vi "Output Enable Write Single.vi"() -> ()   [LabVIEW 2023, in "Output Enable.lvclass"]
uses:
  Output Enable.lvclass
  Output Enable.lvclass/Output Enable.ctl
  <vilib>/ADAS Replay HIL/Channels/Tag Wrapper/Tag Wrapper.lvlib
  <vilib>/ADAS Replay HIL/Channels/Tag Wrapper/Polymorphic/Write Channel (I32).vi
panel:
  in  "Timeout (ms)":i32
  in  "Value to Write":i32
  out "Output Enable out":refnum<class "Output Enable.lvclass">
  in  "Output Enable in":refnum<class "Output Enable.lvclass">
  in  "Channel Index":i32=1
  out "error out":errorcluster
  in  "error in":errorcluster
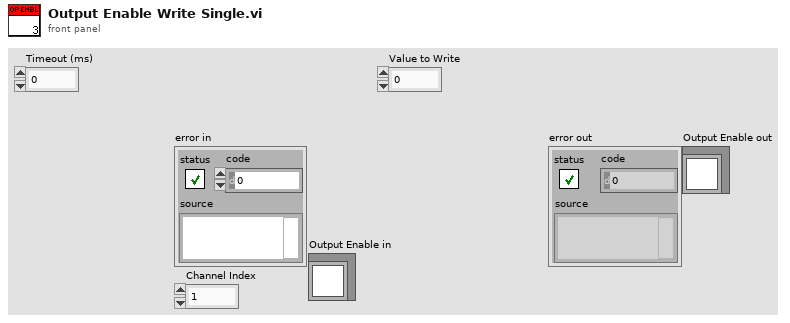
[diagram p1: front panel]
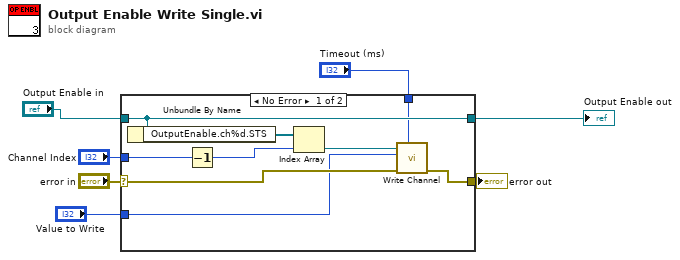
[diagram p0: block diagram]
diagram:
  n1 = case shown="No Error" "error in" {
    selector: "error in" -> [w16 w17]
    tunnel: [w15 w17] -> w6
    tunnel: [w12 w18] -> w3
    tunnel: "Output Enable in" -> [w12 w18]
    tunnel: "Channel Index" -> [w14 _]
    tunnel: "Value to Write" -> [w9 _]
    tunnel: "Timeout (ms)" -> [w8 _]
    frame No Error {
      n2 = Unbundle By Name(w12) -> ("OutputEnable.ch%d.STS"=w11:refnum<k21>[])
      n3 = Decrement(x=w14) -> (x-1=w13:i32)
      n4 = Index Array(array=w11, index=w13) -> (element=w10:refnum<k21>)
      n5 = call-poly <vilib>:"Write Channel.vi"("Timeout (ms)"=w8, "error in"=w16, "Value to Write"=w9, "ADAS HIL Channel in"=w10) -> ("error out"=w15:errorcluster)  [unwired: 5 in, 2 out]
    }
    frame Error {
    }
  }
  "error out" <- w6
  "Output Enable out" <- w3
